vi "_simulator_syncPoint.vi"   [LabVIEW 2011, in "EPS_Timekeeper.lvlib"]
uses:
  <vilib>/addons/Electrical Power/Example Support/PMU/Time Keeper/EPS_Timekeeper.lvlib
types:
  T1 = typedef "Rendezvous RefNum" = refnum<k1>
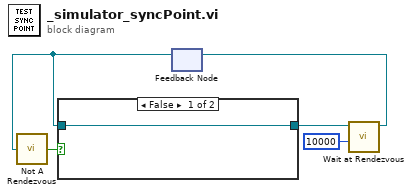
[diagram p0: block diagram]
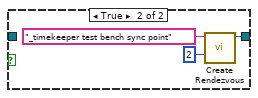
[diagram p2: hidden frame]
diagram:
  n1 = feedback #1() -> (w4:T1)  [unwired: 1 in]
  n2 = call <vilib>:"Not A Rendezvous.vi"("rendezvous"=w4) -> ("not a rendezvous"=w3:bool)
  n3 = case shown="False" w3 {
    tunnel: [w6 w8] -> w5
    tunnel: w4 -> [w6 _]
    frame False {
    }
    frame True {
      n4 = call <vilib>:"Create Rendezvous.vi"("size (2)"=2, "name (unnamed)"="_timekeeper test bench sync point") -> ("rendezvous"=w8:T1)  [unwired: 3 in, 2 out]
    }
  }
  n5 = call <vilib>:"Wait at Rendezvous.vi"("ms timeout (-1)"=10000, "rendezvous"=w5) -> ("rendezvous out"=w2:T1)  [unwired: 3 in, 2 out]
  n6 = feedback-in #1(w2) -> ()
